vi "GetSweepProperties.vi"(9 "channel":string, 10 "data group channels":T12[](array[typedef]), 11 "asset nodes":T1[](array[typedef])) -> (0 "full scale voltage":dbl, 1 "DetectionMode":enum16{"Peak", "Quasi Peak", "Average"}(ring), 2 "detection time":dbl, 3 "sweep freq list":cluster{"frequency":dbl, "bandwidth":dbl}[](array[cluster]), 4 "total number of sweep points":i32)   [LabVIEW 2017, in "EmsaAcquisition.lvlib"]
uses:
  <vilib>/addons/InsightCM/Devices/Shared/Emsa/EmsaAcquisition/EmsaAcquisition.lvlib
  <vilib>/addons/InsightCM/MessageBus/Base/controls/R2_Channel.ctl
  <vilib>/addons/InsightCM/MessageBus/Base/controls/KeyValuePair.ctl
  <vilib>/addons/InsightCM/MessageBus/Base/controls/Metric.ctl
  <vilib>/addons/InsightCM/MessageBus/Base/controls/AssetNode.ctl
  <vilib>/addons/InsightCM/MessageBus/Base/controls/AssetState.ctl
  <vilib>/addons/InsightCM/MessageBus/Base/controls/OperatingState.ctl
  <vilib>/addons/InsightCM/MessageBus/Base/controls/Trigger.ctl
  <vilib>/addons/InsightCM/MessageBus/Base/controls/Condition.ctl
  <vilib>/addons/InsightCM/MessageBus/Base/controls/TrendAlarmRule.ctl
  <vilib>/addons/InsightCM/MessageBus/Base/controls/TrendAlarmLevel.ctl
  <vilib>/addons/InsightCM/MessageBus/Base/controls/AlarmAction.ctl
  <vilib>/addons/InsightCM/MessageBus/Base/controls/AssetNodeReference.ctl
  <vilib>/addons/InsightCM/Utilities/PropertyHelpers/PropertyHelpers.lvlib
  <vilib>/addons/InsightCM/Utilities/DeviceModelHelpers/DeviceModelHelpers.lvlib
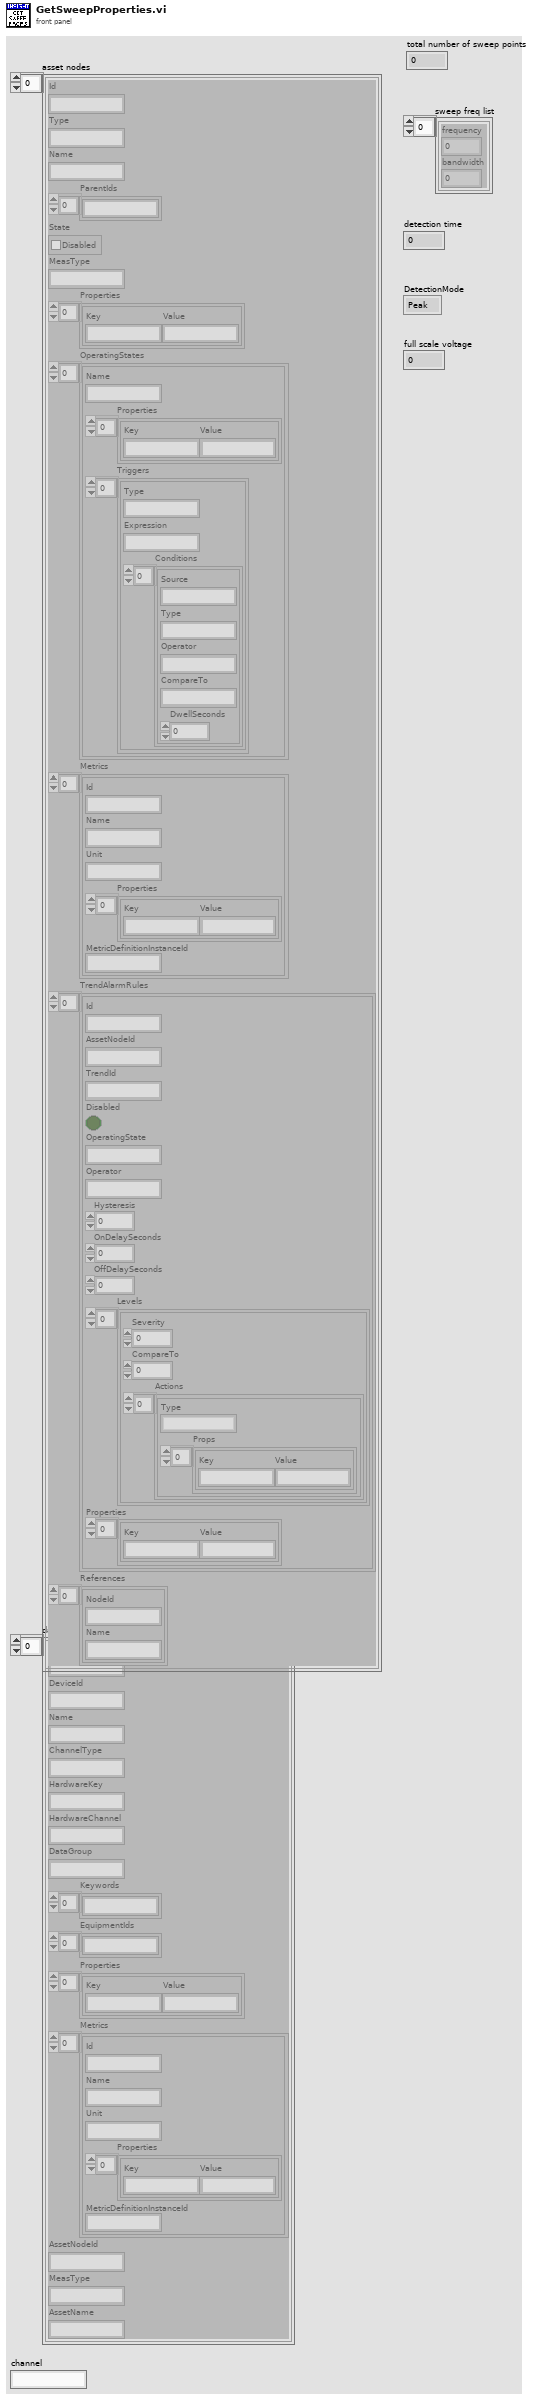
[diagram p1: front panel]
types:
  T1 = typedef "AssetNode.ctl" = cluster{"Id":string, "Type":string, "Name":string, "ParentIds":string[], "State":T2, "MeasType":string, "Properties":T3[], "OperatingStates":T4[], "Metrics":T7[], "TrendAlarmRules":T8[], "References":T11[]}
  T2 = typedef "AssetState.ctl" = cluster{"Disabled":bool}
  T3 = typedef "KeyValuePair.ctl" = cluster{"Key":string, "Value":string}
  T4 = typedef "OperatingState.ctl" = cluster{"Name":string, "Properties":T3[], "Triggers":T5[]}
  T5 = typedef "Trigger.ctl" = cluster{"Type":string, "Expression":string, "Conditions":T6[]}
  T6 = typedef "Condition.ctl" = cluster{"Source":string, "Type":string, "Operator":string, "CompareTo":string, "DwellSeconds":dbl}
  T7 = typedef "Metric.ctl" = cluster{"Id":string, "Name":string, "Unit":string, "Properties":T3[], "MetricDefinitionInstanceId":string}
  T8 = typedef "TrendAlarmRule.ctl" = cluster{"Id":string, "AssetNodeId":string, "TrendId":string, "Disabled":bool, "OperatingState":string, "Operator":string, "Hysteresis":dbl, "OnDelaySeconds":dbl, "OffDelaySeconds":dbl, "Levels":T9[], "Properties":T3[]}
  T9 = typedef "TrendAlarmLevel.ctl" = cluster{"Severity":i32, "CompareTo":dbl, "Actions":T10[]}
  T10 = typedef "AlarmAction.ctl" = cluster{"Type":string, "Props":T3[]}
  T11 = typedef "AssetNodeReference.ctl" = cluster{"NodeId":string, "Name":string}
  T12 = typedef "R2_Channel.ctl" = cluster{"Id":string, "DeviceId":string, "Name":string, "ChannelType":string, "HardwareKey":string, "HardwareChannel":string, "DataGroup":string, "Keywords":string[], "EquipmentIds":string[], "Properties":T3[], "Metrics":T7[], "AssetNodeId":string, "MeasType":string, "AssetName":string}
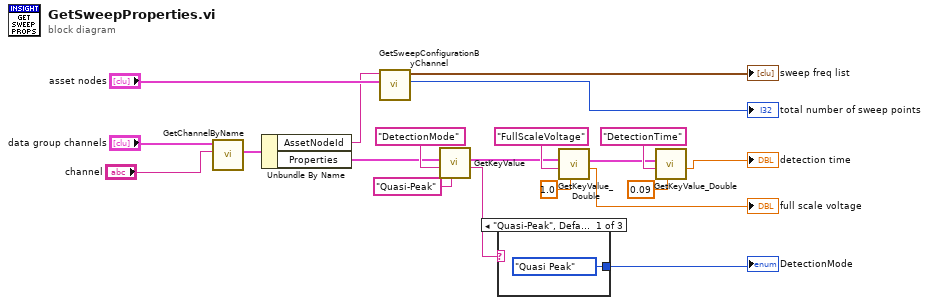
[diagram p0: block diagram]
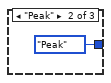
[diagram p2: hidden frame]
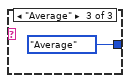
[diagram p3: hidden frame]
diagram:
  n1 = call <vilib>:"GetChannelByName.vi"("channel name"="channel", "channels in"="data group channels") -> ("channel"=w19:T12)  [unwired: 7 in, 2 out]
  n2 = Unbundle By Name(w19) -> ("AssetNodeId"=w16:string, "Properties"=w2:T3[])
  n3 = call <vilib>:"GetSweepConfigurationByChannel.vi"("AssetNodes"="asset nodes", "AssetNodeId"=w16) -> ("total number of points"=→"total number of sweep points":i32, "sweep freq list"=→"sweep freq list":cluster{"frequency":dbl, "bandwidth":dbl}[])  [unwired: 8 in]
  n4 = call <vilib>:"GetKeyValue.vi"("default value"="Quasi-Peak", "key"="DetectionMode", "key value pairs"=w2) -> ("value"=w13:string, "key value pairs out"=w5:T3[])  [unwired: 6 in, 1 out]
  n5 = case shown="\"Quasi-Peak\", Default" w13 {
    tunnel: [enum16{"Peak", "Quasi Peak", "Average"}."Quasi Peak" ("DetectionMode") enum16{"Peak", "Quasi Peak", "Average"}."Peak" ("DetectionMode") enum16{"Peak", "Quasi Peak", "Average"}."Average" ("DetectionMode")] -> w14
    frame "Quasi-Peak", Default {
    }
    frame "Peak" {
    }
    frame "Average" {
    }
  }
  "DetectionMode" <- w14
  n6 = call <vilib>:"GetKeyValue_Double.vi"("default"=1.0, "key"="FullScaleVoltage", "key value pairs"=w5) -> ("value"=→"full scale voltage":dbl, "key value pairs out"=w8:T3[])  [unwired: 6 in, 1 out]
  n7 = call <vilib>:"GetKeyValue_Double.vi"("default"=0.09, "key"="DetectionTime", "key value pairs"=w8) -> ("value"=→"detection time":dbl)  [unwired: 6 in, 2 out]
